vi "Get Request Type.vi"(8 "error in (no error)":errorcluster, 11 "TriggerHotkeyByName in":refnum<class "TriggerHotkeyByName.lvclass">) -> (0 "error out":errorcluster, 2 "Request Type":string, 3 "TriggerHotkeyByName out":refnum<class "TriggerHotkeyByName.lvclass">)   [LabVIEW 2020, in "obs-websocket.lvlib" / "TriggerHotkeyByName.lvclass"]
uses:
  TriggerHotkeyByName.lvclass
  TriggerHotkeyByName.lvclass/TriggerHotkeyByName.ctl
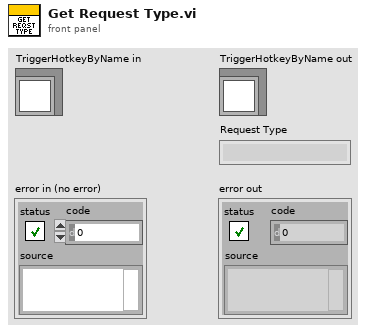
[diagram p1: front panel]
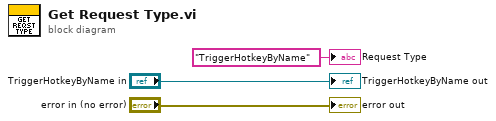
[diagram p0: block diagram]
diagram:
  "error out" <- "error in (no error)"
  "TriggerHotkeyByName out" <- "TriggerHotkeyByName in"
  "Request Type" <- "TriggerHotkeyByName" ("Request Type")
